vi "Get Encoder.vi"() -> (0 "Encoder Data":T1)   [LabVIEW 2018]
uses:
  Encoder Data.ctl
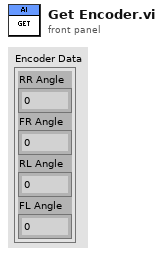
[diagram p1: front panel]
types:
  T1 = typedef "Encoder Data.ctl" = cluster{"RR Angle":dbl, "FR Angle":dbl, "RL Angle":dbl, "FL Angle":dbl}
  T2 = typedef "WPI_AnalogChannelDevRef.ctl" = cluster{"DevStatus":errorcluster, "Analog Channel":T3}
  T3 = typedef "FPGA_AIChannel.ctl" = enum8{"AI 0", "AI 1", "AI 2", "AI 3", "AI MXP 0", "AI MXP 1", "AI MXP 2", "AI MXP 3", "Invalid"}
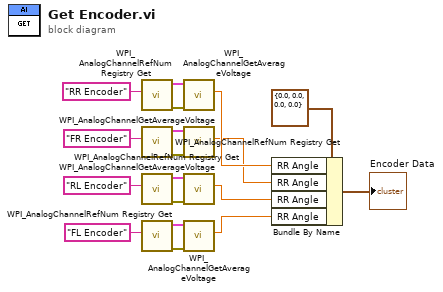
[diagram p0: block diagram]
diagram:
  n1 = call <vilib>:"WPI_AnalogChannelRefNum Registry Get.vi"("refnum name"="RR Encoder") -> ("error out"=w18:errorcluster, "AIDeviceRef"=w17:T2)  [unwired: 9 in]
  n2 = call <vilib>:"WPI_AnalogChannelRefNum Registry Get.vi"("refnum name"="FR Encoder") -> ("error out"=w15:errorcluster, "AIDeviceRef"=w14:T2)  [unwired: 9 in]
  n3 = call <vilib>:"WPI_AnalogChannelRefNum Registry Get.vi"("refnum name"="RL Encoder") -> ("error out"=w12:errorcluster, "AIDeviceRef"=w11:T2)  [unwired: 9 in]
  n4 = call <vilib>:"WPI_AnalogChannelRefNum Registry Get.vi"("refnum name"="FL Encoder") -> ("error out"=w9:errorcluster, "AIDeviceRef"=w8:T2)  [unwired: 9 in]
  n5 = call <vilib>:"WPI_AnalogChannelGetAverageVoltage.vi"("error in (no error)"=w18, "AIDeviceRef"=w17) -> ("Voltage"=w4:dbl)  [unwired: 7 in, 2 out]
  n6 = call <vilib>:"WPI_AnalogChannelGetAverageVoltage.vi"("error in (no error)"=w15, "AIDeviceRef"=w14) -> ("Voltage"=w3:dbl)  [unwired: 7 in, 2 out]
  n7 = call <vilib>:"WPI_AnalogChannelGetAverageVoltage.vi"("error in (no error)"=w12, "AIDeviceRef"=w11) -> ("Voltage"=w2:dbl)  [unwired: 7 in, 2 out]
  n8 = call <vilib>:"WPI_AnalogChannelGetAverageVoltage.vi"("error in (no error)"=w9, "AIDeviceRef"=w8) -> ("Voltage"=w1:dbl)  [unwired: 7 in, 2 out]
  n9 = Bundle By Name(cluster=T1 {"RR Angle"=0.0, "FR Angle"=0.0, "RL Angle"=0.0, "FL Angle"=0.0}, "RR Angle"=w4, "RR Angle"=w3, "RR Angle"=w2, "RR Angle"=w1) -> (→"Encoder Data":T1)
